vi "ConvertGoop2ToGoop3_KeepViPrefix.vi"(1 "OrgViName":path=path "C:/UML/GOOP2/AbstractNode_class/AbstractNode addChild.vi", 2 "ClassFolder":path=path "C:/UML/GOOP2/AbstractNode_class", 5 "error in (no error)":errorcluster, 6 "ClassPrefix":string="AbstractNode ") -> (12 "ClassFolderOut":path, 14 "Don'tUseVI":bool, 15 "KeepPrefix":bool, 16 "NewClassPath":path, 18 "NewClassPathWithPreFix":path, 19 "error out":errorcluster)   [LabVIEW 2014]
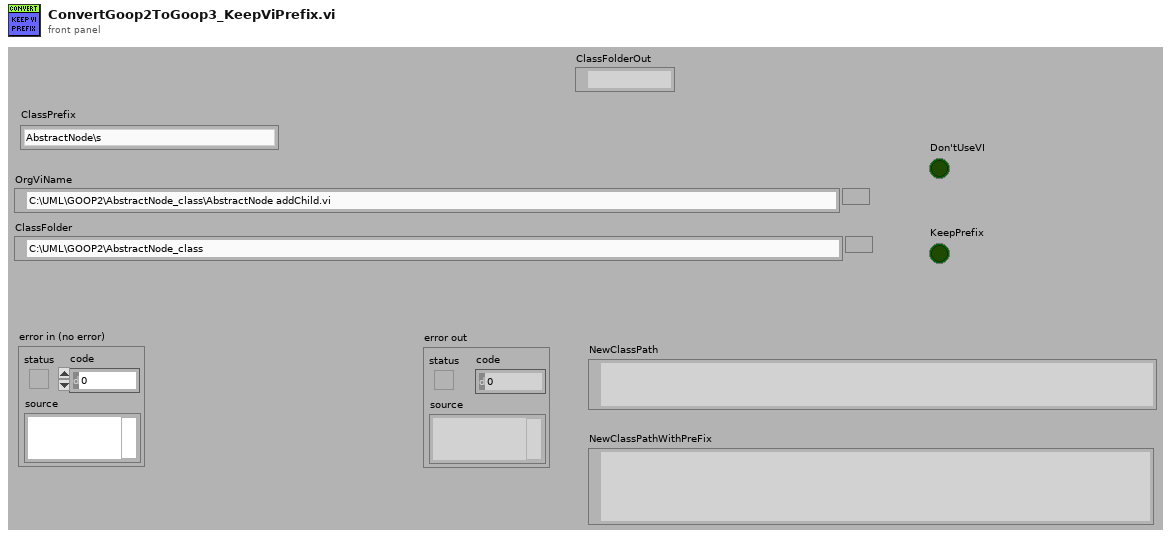
[diagram p1: front panel]
types:
  T1 = typedef "Librarian File Info Out.ctl" = cluster{"creation date":u32, "last mod date":u32, "type":string, "creator":string, "LV version":i32, "size":i32, "top level":bool}
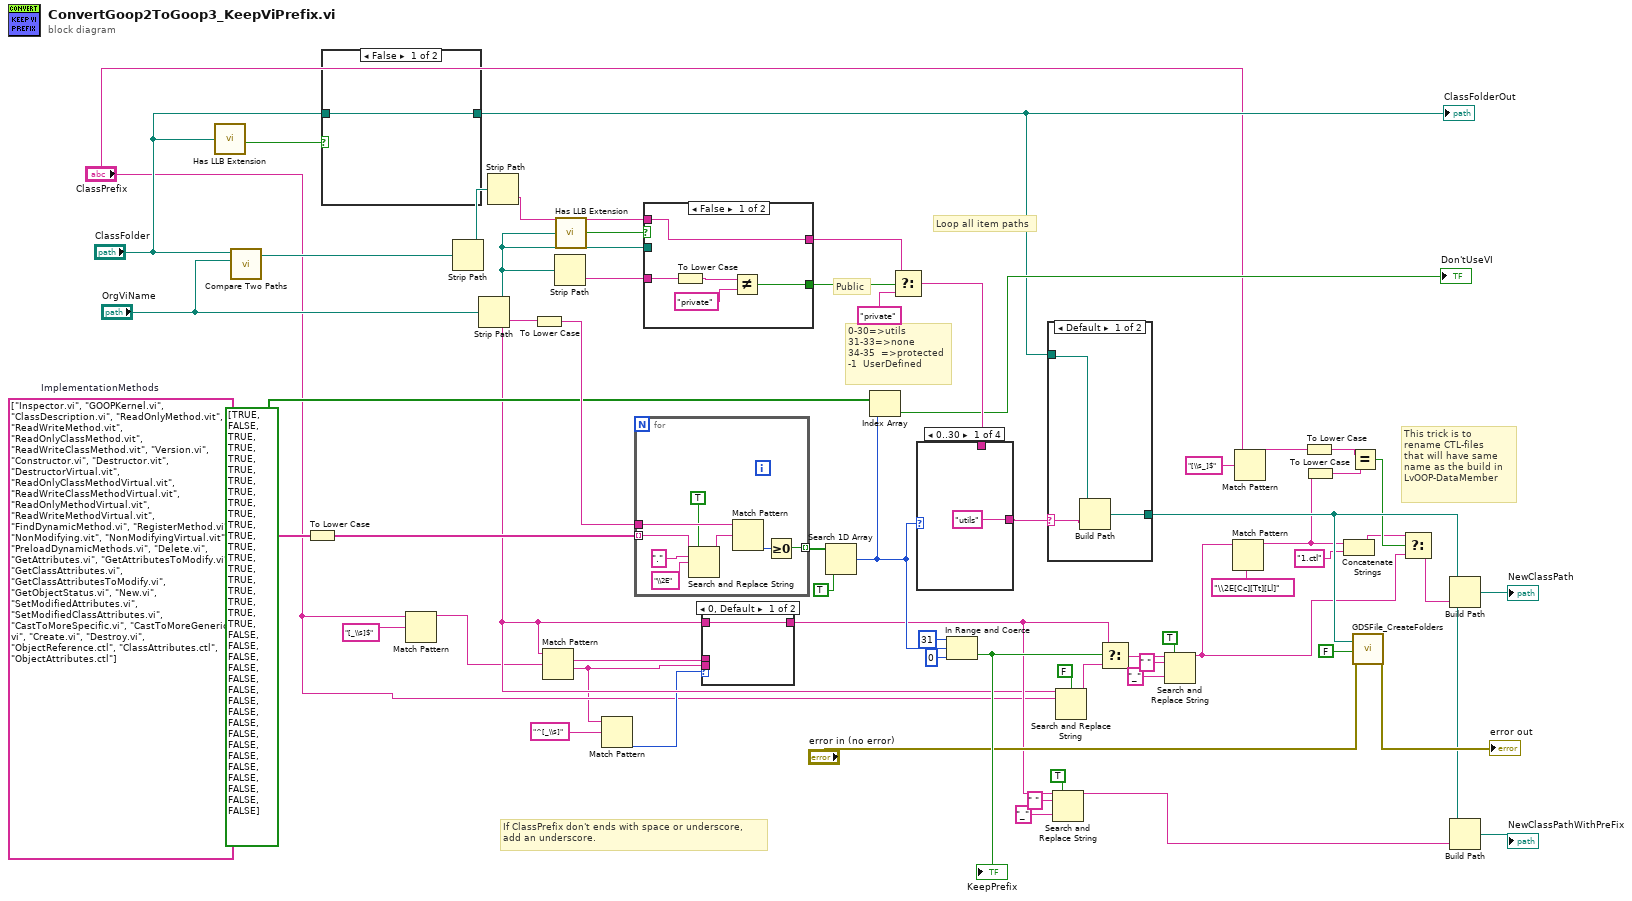
[diagram p0: block diagram]
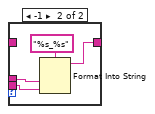
[diagram p2: hidden frame]
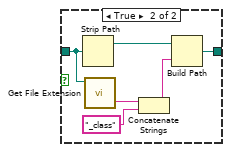
[diagram p3: hidden frame]
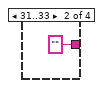
[diagram p5: hidden frame]
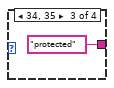
[diagram p6: hidden frame]
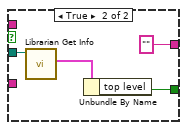
[diagram p8: hidden frame]
diagram:
  w61 = string[] ["Inspector.vi", "GOOPKernel.vi", "ClassDescription.vi", "ReadOnlyMethod.vit", "ReadWriteMethod.vit", "ReadOnlyClassMethod.vit", "ReadWriteClassMethod.vit", "Version.vi", "Constructor.vi", "Destructor.vit", "DestructorVirtual.vit", "ReadOnlyClassMethodVirtual.vit", "ReadWriteClassMethodVirtual.vit", "ReadOnlyMethodVirtual.vit", "ReadWriteMethodVirtual.vit", "FindDynamicMethod.vi", "RegisterMethod.vi", "NonModifying.vit", "NonModifyingVirtual.vit", "PreloadDynamicMethods.vi", "Delete.vi", "GetAttributes.vi", "GetAttributesToModify.vi", "GetClassAttributes.vi", "GetClassAttributesToModify.vi", "GetObjectStatus.vi", "New.vi", "SetModifiedAttributes.vi", "SetModifiedClassAttributes.vi", "CastToMoreSpecific.vi", "CastToMoreGeneric.vi", "Create.vi", "Destroy.vi", "ObjectReference.ctl", "ClassAttributes.ctl", "ObjectAttributes.ctl"]  # ImplementationMethods
  # "If ClassPrefix don't ends with space or underscore,\nadd an underscore."
  # "This trick is to\nrename CTL-files\nthat will have same\nname as the build in\nLvOOP-DataMember"
  # "Public"
  # "0-30=>utils\n31-33=>none\n34-35  =>protected\n-1  UserDefined"
  # "Loop all item paths"
  n1 = call <vilib>:"Has LLB Extension.vi"("path"="ClassFolder") -> ("path to VI library?"=w23:bool)
  n2 = call <vilib>:"Compare Two Paths.vi"("Path 2"="OrgViName", "Path 1"="ClassFolder") -> ("Relative Path from 1 to 2"=w29:path)  [unwired: 6 in, 3 out]
  n3 = To Lower Case(string=w61) -> (all lower case string=w62:string[])
  n4 = case shown="False" w23 {
    tunnel: "ClassFolder" -> [w63 w69]
    tunnel: [w63 w68] -> w21
    frame False {
    }
    frame True {
      n5 = Strip Path(path=w69) -> (stripped path=w65:path)  [unwired: 1 out]
      n6 = call <vilib>:"Get File Extension.vi"("file"=w69) -> ("filename without extension"=w67:string)  [unwired: 7 in, 3 out]
      n7 = Concatenate Strings(w67, "_class" ("string")) -> (w64:string)
      n8 = Build Path(base path=w65, name or relative path=w64) -> (appended path=w68:path)
    }
  }
  "ClassFolderOut" <- w21
  n9 = Match Pattern(string="ClassPrefix", regular expression="[_\\s]$" ("string")) -> (before substring=w3:string)  [unwired: 1 in, 3 out]
  n10 = Strip Path(path=w29) -> (stripped path=w28:path)  [unwired: 1 out]
  n11 = Strip Path(path="OrgViName") -> (stripped path=w58:path, name=w8:string)
  n12 = Strip Path(path=w28) -> (name=w27:string)  [unwired: 1 out]
  n13 = To Lower Case(string=w8) -> (all lower case string=w60:string)
  n14 = Match Pattern(string=w8, regular expression=w3) -> (match substring=w7:string, after substring=w1:string)  [unwired: 1 in, 2 out]
  n15 = Strip Path(path=w58) -> (name=w55:string)  [unwired: 1 out]
  n16 = call <vilib>:"Has LLB Extension.vi"("path"=w58) -> ("path to VI library?"=w59:bool)
  n17 = Match Pattern(string=w1, regular expression="^[_\\s]" ("string")) -> (offset past match=w5:i32)  [unwired: 1 in, 3 out]
  n18 = for {
    tunnel: w62 -> [w76] mode=indexing
    tunnel: w60 -> [w77]
    tunnel: [w70] -> w43 mode=indexing
    n19 = Search and Replace String(replace all?=TRUE ("replace all? (F)"), input string=w76, search string=".", replace string="\\2E" ("replace string (\"\")")) -> (result string=w75:string)  [unwired: 4 in, 3 out]
    n20 = Match Pattern(string=w77, regular expression=w75) -> (offset past match=w71:i32)  [unwired: 1 in, 3 out]
    n21 = Greater Or Equal To 0?(x=w71) -> (x >= 0?=w70:bool)
  }
  n22 = case shown="False" w59 {
    tunnel: w58 -> [_ w86]
    tunnel: w55 -> [w78 _]
    tunnel: [w80 w84] -> w51
    tunnel: [w79 "" ("y")] -> w31
    tunnel: w27 -> [w79 _]
    frame False {
      n23 = To Lower Case(string=w78) -> (all lower case string=w82:string)
      n24 = Not Equal?(x=w82, y="private") -> (x != y?=w80:bool)
    }
    frame True {
      n25 = call <vilib>:"Librarian Get Info.vi"("path"=w86) -> ("file information"=w85:T1)  [unwired: 8 in, 2 out]
      n26 = Unbundle By Name(w85) -> ("top level"=w84:bool)
    }
  }
  n27 = case shown="0, Default" w5 {
    tunnel: w8 -> [w87 _]
    tunnel: [w87 w88] -> w9
    tunnel: w7 -> [_ w90]
    tunnel: w1 -> [_ w89]
    frame 0, Default {
    }
    frame -1 {
      n28 = Format Into String(format string="%s_%s", w90, w89) -> (resulting string=w88:string)  [unwired: 2 in, 1 out]
    }
  }
  n29 = Search 1D Array(1D array=w43, element=TRUE) -> (index of element=w26:i32)  [unwired: 1 in]
  n30 = Index Array(array=bool[] [TRUE, FALSE, TRUE, TRUE, TRUE, TRUE, TRUE, TRUE, TRUE, TRUE, TRUE, TRUE, TRUE, TRUE, TRUE, TRUE, TRUE, TRUE, TRUE, TRUE, FALSE, FALSE, FALSE, FALSE, FALSE, FALSE, FALSE, FALSE, FALSE, FALSE, FALSE, FALSE, FALSE, FALSE, FALSE, FALSE, FALSE] (".not. x?"), index=w26) -> (element=→"Don'tUseVI":bool)
  n31 = Select(t=w31, s=w51, f="private" ("y")) -> (s? t:f=w49:string)
  n32 = case shown="0..30" w26 {
    tunnel: ["utils" "" "protected" w95] -> w48
    tunnel: w49 -> [_ _ _ w95]
    frame 0..30 {
    }
    frame 31..33 {
    }
    frame 34, 35 {
    }
    frame Default {
    }
  }
  n33 = In Range and Coerce(upper limit=31, x=w26, lower limit=0) -> (In Range?=w52:bool)  [unwired: 1 out]
  "KeepPrefix" <- w52
  n34 = case shown="Default" w48 {
    selector: w48 -> [w97 _]
    tunnel: w21 -> [w98 w99]
    tunnel: [w96 w99] -> w38
    frame Default {
      n35 = Build Path(base path=w98, name or relative path=w97) -> (appended path=w96:path)
    }
    frame "" {
    }
  }
  n36 = Search and Replace String(replace all?=TRUE ("replace all? (F)"), input string=w9, search string=" ", replace string="_" ("replace string (\"\")")) -> (result string=w33:string)  [unwired: 4 in, 3 out]
  n37 = Search and Replace String(case sensitive?=FALSE ("ignore case? (F)"), input string=w8, search string="ClassPrefix") -> (result string=w57:string)  [unwired: 5 in, 3 out]
  n38 = Select(t=w9, s=w52, f=w57) -> (s? t:f=w34:string)
  n39 = Search and Replace String(replace all?=TRUE ("replace all? (F)"), input string=w34, search string=" ", replace string="_" ("replace string (\"\")")) -> (result string=w11:string)  [unwired: 4 in, 3 out]
  n40 = Match Pattern(string=w11, regular expression="\\2E[Cc][Tt][Ll]") -> (before substring=w14:string)  [unwired: 1 in, 3 out]
  n41 = Match Pattern(string="ClassPrefix", regular expression="[\\s_]$") -> (before substring=w19:string)  [unwired: 1 in, 3 out]
  n42 = To Lower Case(string=w19) -> (all lower case string=w17:string)
  n43 = To Lower Case(string=w14) -> (all lower case string=w18:string)
  n44 = Concatenate Strings(w14, "1.ctl" ("string")) -> (w12:string)
  n45 = Equal?(x=w17, y=w18) -> (x = y?=w15:bool)
  n46 = call <resource>:"GDSFile_CreateFolders.vi"("Path"=w38, "Promt if folder\ndoes not exists?"=FALSE ("Promt if folder\ndoes not exists?"), "error in (no error)"="error in (no error)") -> ("error out"=→"error out":errorcluster)  [unwired: 12 in, 4 out]
  n47 = Select(t=w12, s=w15, f=w11) -> (s? t:f=w10:string)
  n48 = Build Path(base path=w38, name or relative path=w10) -> (appended path=→"NewClassPath":path)
  n49 = Build Path(base path=w38, name or relative path=w33) -> (appended path=→"NewClassPathWithPreFix":path)
